vi "Day 08 (Part Two).vi"() -> ()   [LabVIEW 2021]
panel:
  out "result":u64
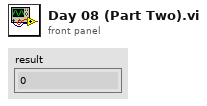
[diagram p1: front panel]
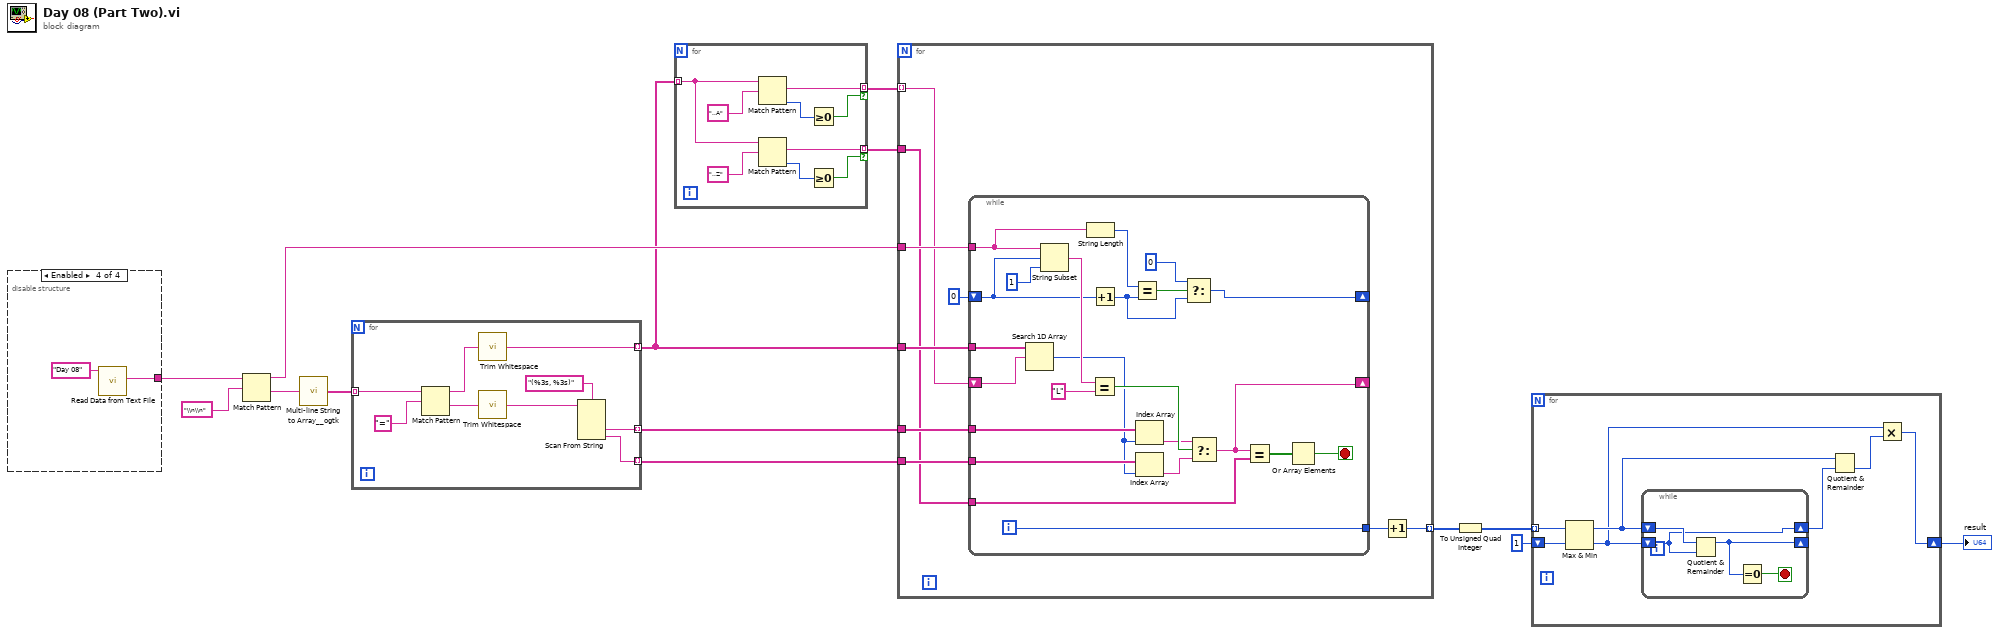
[diagram p0: block diagram]
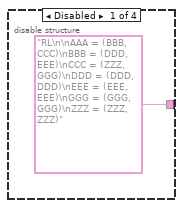
[diagram p2: hidden frame]
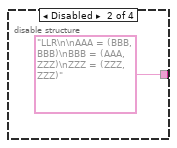
[diagram p3: hidden frame]
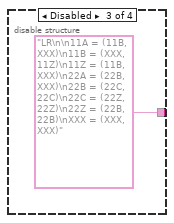
[diagram p4: hidden frame]
diagram:
  n1 = disable-structure shown="Enabled" {
    disable-tunnel: ["RL\n\nAAA = (BBB, CCC)\nBBB = (DDD, EEE)\nCCC = (ZZZ, GGG)\nDDD = (DDD, DDD)\nEEE = (EEE, EEE)\nGGG = (GGG, GGG)\nZZZ = (ZZZ, ZZZ)" "LLR\n\nAAA = (BBB, BBB)\nBBB = (AAA, ZZZ)\nZZZ = (ZZZ, ZZZ)" "LR\n\n11A = (11B, XXX)\n11B = (XXX, 11Z)\n11Z = (11B, XXX)\n22A = (22B, XXX)\n22B = (22C, 22C)\n22C = (22Z, 22Z)\n22Z = (22B, 22B)\nXXX = (XXX, XXX)" w19] -> w4
    frame Disabled {
    }
    frame Disabled {
    }
    frame Disabled {
    }
    frame Enabled {
      n2 = call "Read Data from Text File.vi"("Subfolder"="Day 08") -> ("data"=w19:string)  [unwired: 10 in]
    }
  }
  n3 = Match Pattern(string=w4, regular expression="\\n\\n") -> (before substring=w9:string, after substring=w13:string)  [unwired: 1 in, 2 out]
  n4 = call <userlib>:"Multi-line String to Array__ogtk.vi"("string"=w13) -> ("lines"=w12:string[])
  n5 = for {
    tunnel: w12 -> [w28] mode=indexing
    tunnel: [w22] -> w8 mode=indexing
    tunnel: [w21] -> w11 mode=indexing
    tunnel: [w20] -> w10 mode=indexing
    n6 = Match Pattern(string=w28, regular expression="=") -> (before substring=w26:string, after substring=w25:string)  [unwired: 1 in, 2 out]
    n7 = call <vilib>:"Trim Whitespace.vi"("string"=w26) -> ("trimmed string"=w22:string)  [unwired: 1 in]
    n8 = call <vilib>:"Trim Whitespace.vi"("string"=w25) -> ("trimmed string"=w23:string)  [unwired: 1 in]
    n9 = Scan From String(format string="(%3s, %3s)", input string=w23) -> (output 1=w21:string, output 2=w20:string)  [unwired: 4 in, 3 out]
  }
  n10 = for {
    tunnel: w8 -> [w35] mode=indexing
    tunnel: [w34] -> w7 mode=indexing if=w30
    tunnel: [w33] -> w6 mode=indexing if=w29
    n11 = Match Pattern(string=w35, regular expression="..A") -> (match substring=w34:string, offset past match=w32:i32)  [unwired: 1 in, 2 out]
    n12 = Match Pattern(string=w35, regular expression="..Z") -> (match substring=w33:string, offset past match=w31:i32)  [unwired: 1 in, 2 out]
    n13 = Greater Or Equal To 0?(x=w32) -> (x >= 0?=w30:bool)
    n14 = Greater Or Equal To 0?(x=w31) -> (x >= 0?=w29:bool)
  }
  n15 = for {
    tunnel: w11 -> [w46]
    tunnel: w10 -> [w45]
    tunnel: w9 -> [w42]
    tunnel: w8 -> [w41]
    tunnel: w7 -> [w40] mode=indexing
    tunnel: w6 -> [w39]
    tunnel: [w38] -> w5 mode=indexing
    n16 = while {
      tunnel: w46 -> [w62]
      tunnel: w45 -> [w61]
      shift-right: [w50] -> _
      shift-left: w40 -> [w66]
      tunnel: w41 -> [w67]
      shift-right: [w60] -> _
      shift-left: 0 ("t") -> [w52]
      tunnel: [w56] -> w43
      tunnel: w42 -> [w54]
      tunnel: w39 -> [w49]
      i -> [w56]
      stop <- w47 stop-if-true
      n17 = Search 1D Array(1D array=w67, element=w66) -> (index of element=w51:i32)  [unwired: 1 in]
      n18 = String Subset(string=w54, offset (0)=w52, length (rest)=1 ("length (rest)")) -> (substring=w59:string)
      n19 = String Length(string=w54) -> (length=w53:i32)
      n20 = Equal?(x=w59, y="L") -> (x = y?=w68:bool)
      n21 = Increment(x=w52) -> (x+1=w64:i32)
      n22 = Equal?(x=w53, y=w64) -> (x = y?=w65:bool)
      n23 = Index Array(array=w62, index=w51) -> (element=w58:string)
      n24 = Index Array(array=w61, index=w51) -> (element=w57:string)
      n25 = Select(t=0, s=w65, f=w64) -> (s? t:f=w60:i32)
      n26 = Select(t=w58, s=w68, f=w57) -> (s? t:f=w50:string)
      n27 = Equal?(x=w50, y=w49) -> (x = y?=w48:bool[])
      n28 = Or Array Elements(Boolean array=w48) -> (logical OR=w47:bool)
    }
    n29 = Increment(x=w43) -> (x+1=w38:i32)
  }
  n30 = To Unsigned Quad Integer(1:w5) -> (0:w2:u64[])
  n31 = for {
    tunnel: w2 -> [w72] mode=indexing
    shift-right: [w74] -> w1
    shift-left: u64 1 -> [w73]
    n32 = Max & Min(x=w72, y=w73) -> (max(x,y)=w71:u64, min(x,y)=w70:u64)
    n33 = while {
      shift-right: [w78] -> _
      shift-left: w70 -> [w77]
      shift-right: [w77] -> w75
      shift-left: w71 -> [w79]
      stop <- w80 stop-if-true
      n34 = Quotient & Remainder(x=w79, y=w77) -> (x-y*floor(x/y)=w78:u64)  [unwired: 1 out]
      n35 = Equal To 0?(x=w78) -> (x = 0?=w80:bool)
    }
    n36 = Quotient & Remainder(x=w71, y=w75) -> (floor(x/y)=w76:u64)  [unwired: 1 out]
    n37 = Multiply(x=w70, y=w76) -> (x*y=w74:u64)
  }
  "result" <- w1
